vi "VIPC File -- List Packages__vipm_api_vipm_api.vi"(8 "error in (no error)":errorcluster, 11 "VIPC File Path":path) -> (0 "error out":errorcluster, 1 "VIPC LabVIEW Version":string, 2 "Package List":string[](array[string]), 3 "VIPC File Path (dup)":path)   [LabVIEW 2017, in "VIP SBOM Support.lvlib"]
doc: "Local (public) copy of a private VIPM API VI to retrieve list of packages in a package configuration file (VIPC).\n\nCopyright 2009-2012 JKI\n______________________________________\nVIPM API 2017.0.0.55\nCopyright (c) 2015, JKI. All rights reserved.\n\nThis library is provided \"AS IS\" ,WITHOUT WARRANTIES OR \nCONDITIONS OF ANY KIND, either express or implied.\n\nJKI -- jki.net"
uses:
  VIP SBOM Support.lvlib
  <vilib>/JKI/_VIPM API_internal_deps/ZLIB Open Unzip Archive__ogtk4A668244C627608002181B7F01911EC7.vi
  <vilib>/JKI/_VIPM API_internal_deps/ZLIB Extract Stream__ogtk4A668244C627608002181B7F01911EC7.vi
  <vilib>/zip/NI_Unzip.lvlib
  <userlib>/_OpenG.lib/file/file.llb/Compare Two Paths - Path2 Array__ogtk.vi
  <vilib>/JKI/_VIPM API_internal_deps/Strip Path - Traditional__ogtk4A668244C627608002181B7F01911EC7.vi
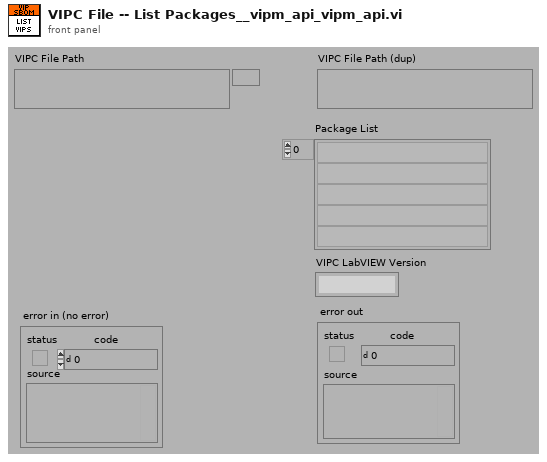
[diagram p1: front panel]
types:
  T1 = typedef "ZLIB Unzip Handle__ogtk4A668244C627608002181B7F01911EC7.ctl" = refnum<k1>
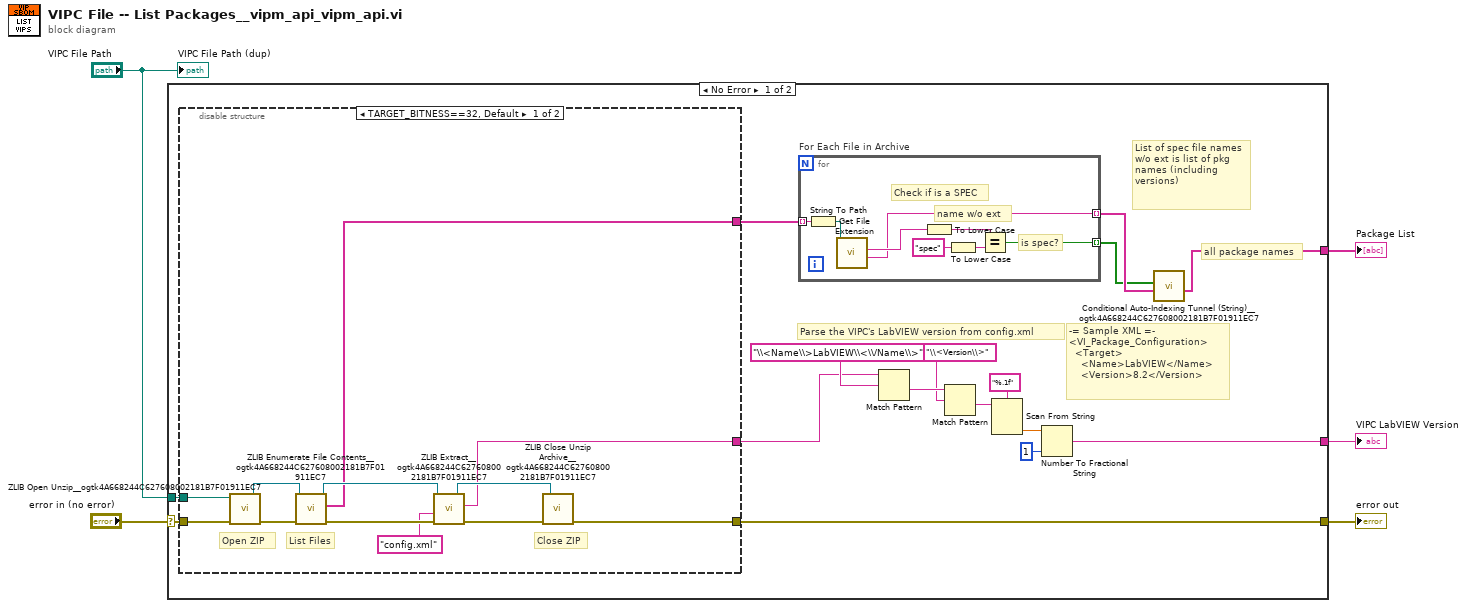
[diagram p0: block diagram]
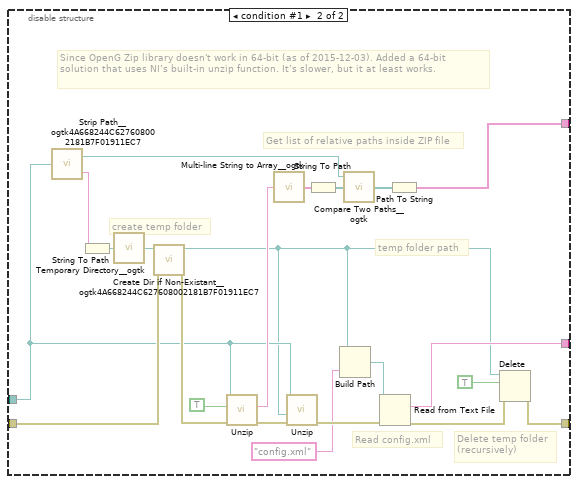
[diagram p2: hidden frame]
diagram:
  n1 = case shown="No Error" "error in (no error)" {
    selector: "error in (no error)" -> [w20 w64]
    tunnel: [w8 _] -> w4
    tunnel: [w19 w64] -> w3
    tunnel: "VIPC File Path" -> [w21 _]
    tunnel: [w7 _] -> w1
    frame No Error {
      # "all package names"
      # "-= Sample XML =-\n<VI_Package_Configuration>\n  <Target>\n    <Name>LabVIEW</Name>\n    <Version>8.2</Version>"
      # "Parse the VIPC's LabVIEW version from config.xml"
      # "List of spec file names w/o ext is list of pkg names (including versions)"
      n2 = disable-structure shown="TARGET_BITNESS==32, Default" {
        disable-tunnel: w21 -> [w39 w49]
        disable-tunnel: w20 -> [w38 w60]
        disable-tunnel: [w33 w46] -> w19
        disable-tunnel: [w32 w53] -> w9
        disable-tunnel: [w31 w51] -> w6
        frame condition #0 (active) {
          # "Close ZIP"
          # "List Files"
          # "Open ZIP"
          n3 = call-poly <vilib>:"ZLIB Open Unzip__ogtk4A668244C627608002181B7F01911EC7.vi"("error in (no error)"=w38, "archive name"=w39) -> ("error out"=w41:errorcluster, "unzip Refnum"=w40:T1)  [unwired: 4 in]
          n4 = call <vilib>:"ZLIB Enumerate File Contents__ogtk4A668244C627608002181B7F01911EC7.vi"("error in (no error)"=w41, "unzip Refnum"=w40) -> ("error out"=w36:errorcluster, "file names"=w32:string[], "unzip Refnum out"=w37:T1)  [unwired: 5 in, 2 out]
          n5 = call-poly <vilib>:"ZLIB Extract__ogtk4A668244C627608002181B7F01911EC7.vi"("error in (no error)"=w36, "internal name"="config.xml" ("extension"), "unzip Refnum"=w37) -> ("error out"=w34:errorcluster, "byte stream"=w31:string, "unzip Refnum out"=w35:T1)  [unwired: 4 in]
          n6 = call <vilib>:"ZLIB Close Unzip Archive__ogtk4A668244C627608002181B7F01911EC7.vi"("error in (no error)"=w34, "unzip Refnum"=w35) -> ("error out"=w33:errorcluster)  [unwired: 5 in]
        }
        frame condition #1 {
          # "Since OpenG Zip library doesn't work in 64-bit (as of 2015-12-03). Added a 64-bit solution that uses NI’s built-in unzip function. It’s slower, but it at least works."
          # "Delete temp folder\n(recursively)"
          # "Read config.xml"
          # "temp folder path"
          # "Get list of relative paths inside ZIP file"
          # "create temp folder"
          n7 = call-poly <vilib>:"Strip Path__ogtk4A668244C627608002181B7F01911EC7.vi"("path"=w49) -> ("stripped path"=w50:path, "name"=w63:string)
          n8 = String To Path(string=w63) -> (path=w62:path)
          n9 = call <userlib>:"Temporary Directory__ogtk.vi"("Relative path (.)"=w62) -> ("Temporary Directory (+ Relative)"=w61:path)
          n10 = call <vilib>:"Create Dir if Non-Existant__ogtk4A668244C627608002181B7F01911EC7.vi"("error in (no error)"=w60, "Directory Path"=w61) -> ("error out"=w59:errorcluster, "dup Directory Path"=w45:path)  [unwired: 7 in, 1 out]
          n11 = call <vilib>:"Unzip.vi"("error in (no error)"=w59, "Preview only?"=TRUE, "Zip file"=w49) -> ("error out"=w48:errorcluster, "Preview"=w57:string)  [unwired: 6 in, 1 out]
          n12 = call <userlib>:"Multi-line String to Array__ogtk.vi"("string"=w57) -> ("lines"=w56:string[])
          n13 = call <vilib>:"Unzip.vi"("error in (no error)"=w48, "Target directory (same as Zip file if empty)"=w45, "Zip file"=w49) -> ("error out"=w47:errorcluster)  [unwired: 6 in, 2 out]
          n14 = String To Path(string=w56) -> (path=w55:path[])
          n15 = Build Path(base path=w45, name or relative path="config.xml" ("extension")) -> (appended path=w52:path)
          n16 = call-poly <userlib>:"Compare Two Paths__ogtk.vi"("path2"=w55, "path1"=w50) -> ("relative path from 1 to 2"=w54:path[])  [unwired: 1 in, 2 out]
          n17 = Read from Text File(file (use dialog)=w52, error in=w47) -> (text=w51:string, error out=w42:errorcluster)  [unwired: 2 in, 2 out]
          n18 = Path To String(path=w54) -> (string=w53:string[])
          n19 = Delete(path (use dialog)=w45, entire hierarchy (F)=TRUE, error in=w42) -> (error out=w46:errorcluster)  [unwired: 2 in, 2 out]
        }
      }
      n20 = for "For Each File in Archive" {
        tunnel: w9 -> [w25] mode=indexing
        tunnel: [w26] -> w17 mode=indexing
        tunnel: [w23] -> w18 mode=indexing
        # "is spec?"
        # "name w/o ext"
        # "Check if is a SPEC"
        n21 = String To Path(string=w25) -> (path=w22:path)
        n22 = call <vilib>:"Get File Extension.vi"("file"=w22) -> ("filename without extension"=w23:string, "lowercase file extension"=w24:string)  [unwired: 6 in, 3 out]
        n23 = To Lower Case(string=w24) -> (all lower case string=w28:string)
        n24 = To Lower Case(string="spec" ("extension")) -> (all lower case string=w27:string)
        n25 = Equal?(x=w28, y=w27) -> (x = y?=w26:bool)
      }
      n26 = Match Pattern(string=w6, regular expression="\\<Name\\>LabVIEW\\<\\/Name\\>") -> (after substring=w12:string)  [unwired: 1 in, 3 out]
      n27 = Match Pattern(string=w12, regular expression="\\<Version\\>") -> (after substring=w15:string)  [unwired: 1 in, 3 out]
      n28 = Scan From String(format string="%.1f", input string=w15) -> (output 1=w14:dbl)  [unwired: 3 in, 3 out]
      n29 = Number To Fractional String(number=w14, precision (6)=i16 1) -> (F-format string=w7:string)  [unwired: 2 in]
      n30 = call <vilib>:"Conditional Auto-Indexing Tunnel (String)__ogtk4A668244C627608002181B7F01911EC7.vi"("Array in"=w18, "Elements to keep"=w17) -> ("Filtered Array out"=w8:string[])  [unwired: 5 in]
    }
    frame Error {
    }
  }
  "error out" <- w3
  "Package List" <- w4
  "VIPC LabVIEW Version" <- w1
  "VIPC File Path (dup)" <- "VIPC File Path"
